vi "FTW-ProjectItemManager-TransactionQueue-RemoveFromWrite.vi"(0 "Project Item Manager":refnum<class "FTW-ProjectItemManager.lvclass">, 5 "Tag Regex to Match":string, 7 "Force Literal Match?":bool, 11 "error in":errorcluster) -> (4 "Project Item Manager out":refnum<class "FTW-ProjectItemManager.lvclass">, 15 "error out":errorcluster)   [LabVIEW 2012, in "FTW-ProjectItemManager.lvclass"]
uses:
  FTW-ProjectItemManager.lvclass
  FTW-ProjectItemManager.lvclass/FTW-ProjectItemManager.ctl
panel:
  # "Inputs"
  # "Outputs"
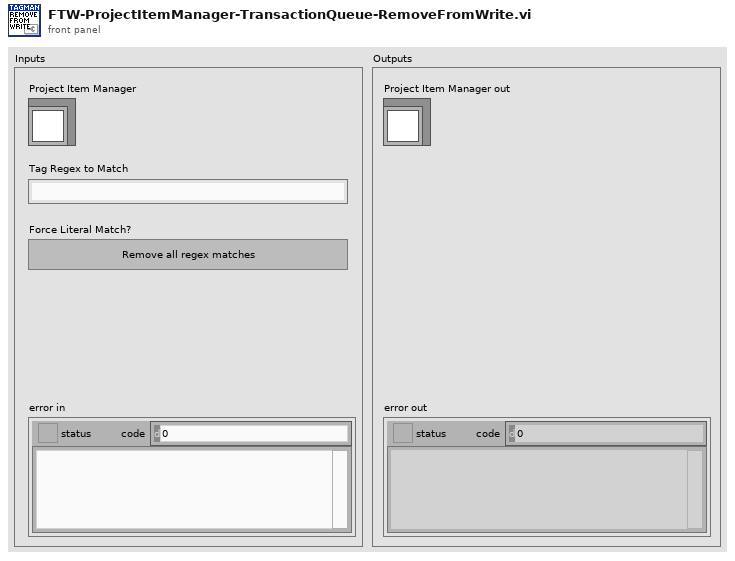
[diagram p1: front panel]
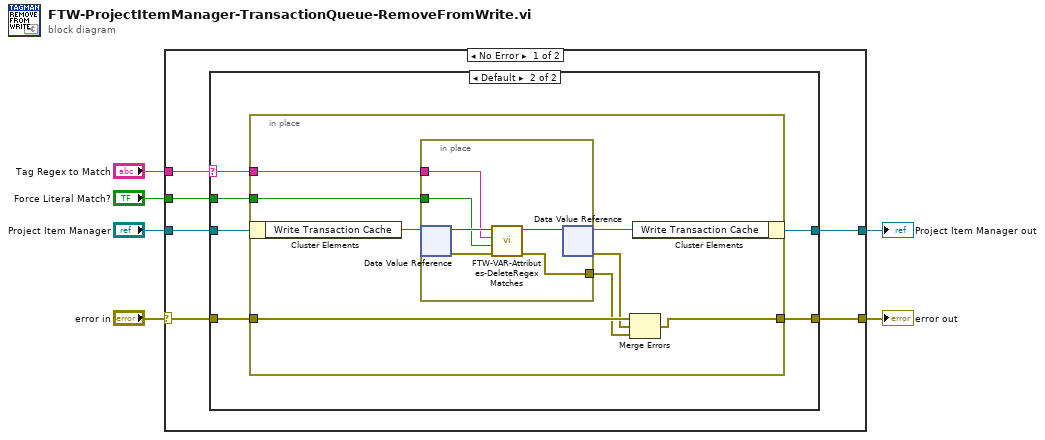
[diagram p0: block diagram]
diagram:
  n1 = case shown="No Error" "error in" {
    selector: "error in" -> [w12 w36]
    tunnel: [w11 w36] -> w6
    tunnel: [w9 w35] -> w4
    tunnel: "Project Item Manager" -> [w10 w35]
    tunnel: "Tag Regex to Match" -> [w8 _]
    tunnel: "Force Literal Match?" -> [w7 _]
    frame No Error {
      n2 = case shown="Default" w8 {
        selector: w8 -> [_ w20]
        tunnel: w12 -> [w13 w18]
        tunnel: [w13 w15] -> w11
        tunnel: w10 -> [w14 w17]
        tunnel: [w14 w16] -> w9
        tunnel: w7 -> [_ w19]
        frame "" {
        }
        frame Default {
          n3 = in-place {
            in-place-border: [w28] -> w15
            in-place-border: w20 -> [w27]
            in-place-border: w19 -> [w26]
            in-place-border: w18 -> [w25]
            n4 = in-place-cluster #1(w17) -> ("Write Transaction Cache"=w22:refnum<data-value>)
            n5 = in-place {
              in-place-border: [w29] -> w23
              in-place-border: w27 -> [w32]
              in-place-border: w26 -> [w31]
              n6 = in-place-dvr #2(w22) -> (w34:variant, w33:errorcluster)
              n7 = call "FTW-VAR-Attributes-DeleteRegexMatches.vi"("error in"=w33, "Force Literal Match?"=w31, "Regex Match for Attributes"=w32, "Variant"=w34) -> ("error out"=w29:errorcluster, "Variant out"=w30:variant)  [unwired: 4 in, 2 out]
              n8 = in-place-dvr #2(w30) -> (w21:refnum<data-value>, w24:errorcluster)
            }
            n9 = Merge Errors(w25, w24, w23) -> (w28:errorcluster)
            n10 = in-place-cluster #1("Write Transaction Cache"=w21) -> (w16:refnum<class "FTW-ProjectItemManager.lvclass">)
          }
        }
      }
    }
    frame Error {
    }
  }
  "error out" <- w6
  "Project Item Manager out" <- w4
